vi "Get Read Position.vi"(8 "error in (no error)":errorcluster, 11 "FileStream in":refnum<class "FileStream.lvclass">) -> (0 "error out":errorcluster, 2 "Read Position":i64, 3 "FileStream out":refnum<class "FileStream.lvclass">)   [LabVIEW 2020, in "IO.lvlib" / "FileStream.lvclass"]
uses:
  FileStream.lvclass
  FileStream.lvclass/FileStream.ctl
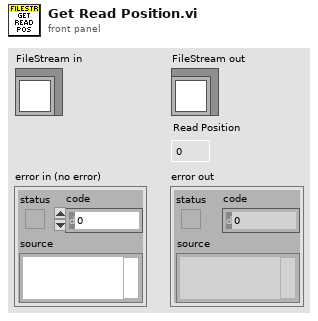
[diagram p1: front panel]
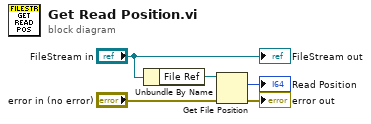
[diagram p0: block diagram]
diagram:
  n1 = Unbundle By Name("FileStream in") -> ("File Ref"=w5:refnum<file>)
  n2 = Get File Position(4:"error in (no error)", 7:w5) -> (0:→"error out":errorcluster, 2:→"Read Position":i64)  [unwired: 1 out]
  "FileStream out" <- "FileStream in"
